vi "Spreadsheet Example.vi"() -> ()   [LabVIEW 2018]
doc: "이 VI는 LabVIEW Core 1 교육 과정의 연습문제입니다.\n\n이 VI는 3개의 데이터 배열을 생성한 후 2D 배열로 결합하여 그래프로 나타내며, [스프레드시트 파일에 쓰기]라는 이름의 상위 레벨 파일 I/O 함수를 사용하여 해당 2D 배열 데이터를 스프레드시트 형식의 파일로 씁니다."
uses:
  <vilib>/Utility/file.llb/Write To Spreadsheet File (DBL).vi
  <vilib>/Analysis/NI_AALBase.lvlib
panel:
  out "테이블":string[][](table)
  out "웨이브폼 그래프":dbl[][](graph)
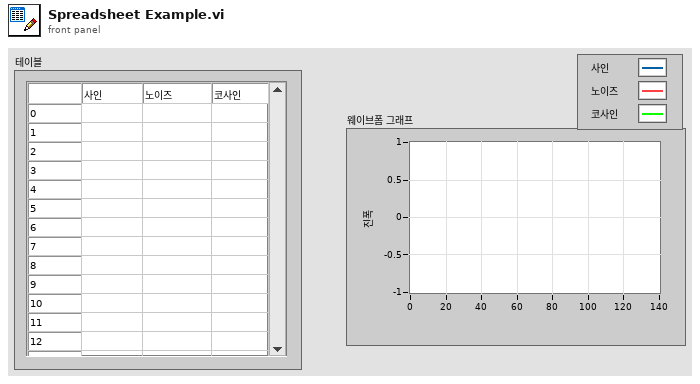
[diagram p1: front panel]
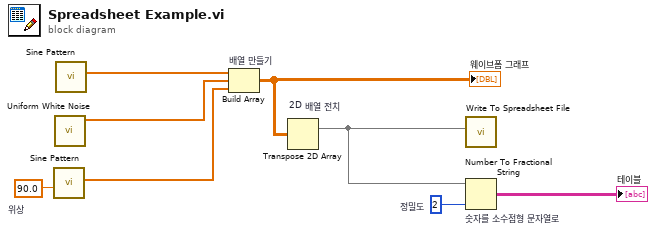
[diagram p0: block diagram]
diagram:
  w5 = 2  # 정밀도
  w6 = 90.0  # 위상
  n1 = call <vilib>:"Sine Pattern.vi"("phase(degrees)"=w6) -> ("Sinusoidal Pattern"=w3:dbl[])  [unwired: 3 in, 1 out]
  n2 = call <vilib>:"Uniform White Noise.vi"() -> ("uniform white noise"=w8:dbl[])  [unwired: 10 in, 1 out]
  n3 = call <vilib>:"Sine Pattern.vi"() -> ("Sinusoidal Pattern"=w7:dbl[])  [unwired: 4 in, 1 out]
  n4 = Build Array "배열 만들기"(w7, w8, w3) -> (w1:dbl[][])
  "웨이브폼 그래프" <- w1
  n5 = Transpose 2D Array "2D 배열 전치"(2D array=w1) -> (transposed array=w4:dbl[][])
  n6 = call-poly <vilib>:"Write To Spreadsheet File.vi"("2D data"=w4) -> ()  [unwired: 7 in, 1 out]
  n7 = Number To Fractional String "숫자를 소수점형 문자열로"(number=w4, precision (6)=w5) -> (F-format string=→"테이블":string[][])  [unwired: 2 in]
